vi "FVI_Motor_1Vitessecercle.vi"(11 "Axe R X":dbl) -> (1 "ARD":dbl, 2 "AVG":dbl, 3 "AVD":dbl, 4 "ARG":dbl)   [LabVIEW 2018]
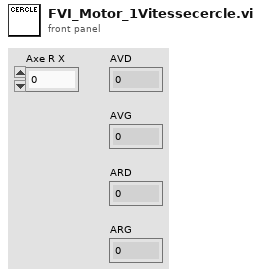
[diagram p1: front panel]
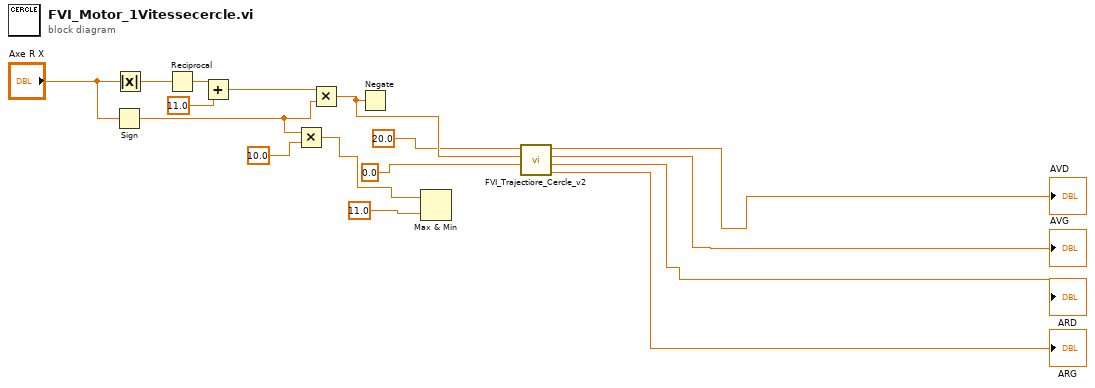
[diagram p0: block diagram]
diagram:
  n1 = Sign(1:"Axe R X") -> (0:w3:dbl)
  n2 = Absolute Value(x="Axe R X") -> (abs(x)=w2:dbl)
  n3 = Reciprocal(x=w2) -> (1/x=w13:dbl)
  n4 = Add(x=w13, y=11.0) -> (x+y=w15:dbl)
  n5 = Multiply(x=w3, y=10.0 ("Rayon x")) -> (x*y=w11:dbl)
  n6 = Multiply(x=w15, y=w3) -> (x*y=w16:dbl)
  n7 = Negate(x=w16) -> ()  [unwired: 1 out]
  n8 = Max & Min(x=w11, y=11.0 ("Rayon x")) -> ()  [unwired: 2 out]
  n9 = call "FVI_Trajectiore_Cercle_v2.vi"("Rayon y"=0.0, "Rayon x"=w16, "dst"=20.0) -> ("ARG"=→"ARG":dbl, "ARD"=→"ARD":dbl, "AVG"=→"AVG":dbl, "AVD"=→"AVD":dbl)  [unwired: 5 in]
